vi "p1.vi"() -> ()   [LabVIEW 2021, in "d3.lvlib"]
uses:
  d3.lvlib
  <vilib>/regexp/Match Regular Expression.xnode
  AOC/AOC.lvlib
panel:
  in  "Example":string="vJrwpWtwJgWrhcsFMMfFFhFp\njqHRNqRjqzjGDLGLrsFMfFZSrLrFZsSL\nPmmdzqPrVvPwwTWBwg\nwMqvLMZHhHMvwLHjbvcjnnSBnvTQFn\nttgJtRGJQctTZtZT\nCrZsJsPPZsGzwwsLwLmpwMDw"
  in  "Example":bool
  out "Answer":i64=7746
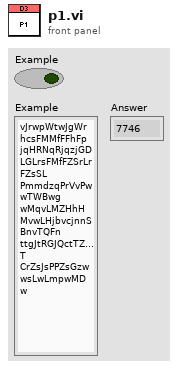
[diagram p1: front panel]
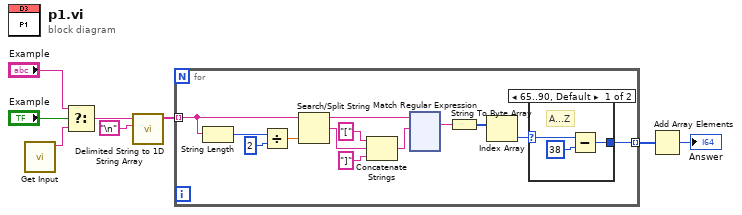
[diagram p0: block diagram]
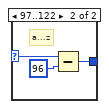
[diagram p2: hidden frame]
diagram:
  n1 = call "Get Input.vi"() -> ("Input"=w6:string)  [unwired: 11 in]
  n2 = Select(t="Example", s="Example", f=w6) -> (s? t:f=w5:string)
  n3 = call <vilib>:"Delimited String to 1D String Array.vi"("delimiter"="\n", "delimited string"=w5) -> ("string array"=w3:string[])  [unwired: 9 in]
  n4 = for {
    tunnel: w3 -> [w21] mode=indexing
    tunnel: [w9] -> w7 mode=indexing
    n5 = String Length(string=w21) -> (length=w20:i32)
    n6 = Divide(x=w20, y=2) -> (x/y=w19:dbl)
    n7 = Search/Split String(string=w21, offset (0)=w19) -> (substring before match=w17:string, match + rest of string=w16:string)  [unwired: 1 in, 1 out]
    n8 = Concatenate Strings("[" ("string"), w16, "]" ("string")) -> (w15:string)
    n9 = xnode "Match Regular Expression"("input string"=w17, "regular expression"=w15) -> ("whole match"=w12:string)  [unwired: 4 in, 4 out]
    n10 = String To Byte Array(string=w12) -> (unsigned byte array=w11:u8[])
    n11 = Index Array(array=w11) -> (element=w10:u8)  [unwired: 1 in]
    n12 = case shown="65..90, Default" w10 {
      selector: w10 -> [w24 w27]
      tunnel: [w22 w25] -> w9
      frame 65..90, Default {
        # "A...Z"
        n13 = Subtract(x=w24, y=u64 38) -> (x-y=w22:u64)
      }
      frame 97..122 {
        # "a...z"
        n14 = Subtract(x=w27, y=u8 96) -> (x-y=w25:u8)
      }
    }
  }
  n15 = Add Array Elements(numeric array=w7) -> (sum=→"Answer":u64)
